vi "Write Size (Bounding Rect).vi"(8 "error in (no error)":errorcluster, 10 "Size (Bounding Rect)":T1, 11 "UI Object in":refnum<class "UI Object.lvclass">) -> (0 "error out":errorcluster, 3 "UI Object out":refnum<class "UI Object.lvclass">)   [LabVIEW 2016, in "PacManClasses.lvlib" / "UI Object.lvclass"]
uses:
  UI Object.lvclass
  Generic Controls/Size - Bounding Rect.ctl
  UI Object.lvclass/UI Object.ctl
  PacManClasses.lvlib
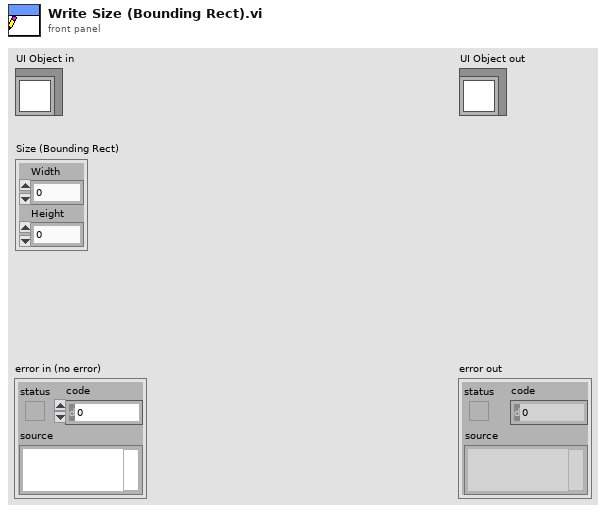
[diagram p1: front panel]
types:
  T1 = typedef "PacManClasses.lvlib/Size - Bounding Rect.ctl" = cluster{"Width":u16, "Height":u16}
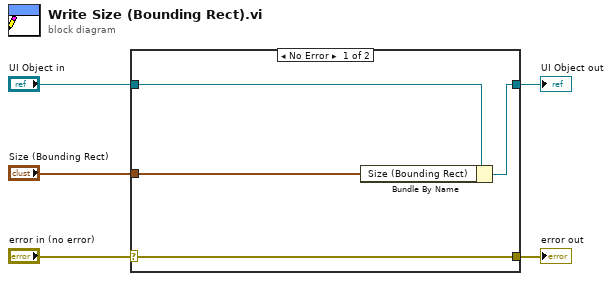
[diagram p0: block diagram]
diagram:
  n1 = case shown="No Error" "error in (no error)" {
    selector: "error in (no error)" -> [w9 w10]
    tunnel: [w9 w10] -> w4
    tunnel: [w7 w11] -> w2
    tunnel: "UI Object in" -> [w8 w11]
    tunnel: "Size (Bounding Rect)" -> [w6 _]
    frame No Error {
      n2 = Bundle By Name(cluster=w8, "Size (Bounding Rect)"=w6) -> (w7:refnum<class "UI Object.lvclass">)
    }
    frame Error {
    }
  }
  "error out" <- w4
  "UI Object out" <- w2
